vi "Get Library Icon.vi"(8 "error in (no error)":errorcluster, 11 "Library Refnum in":refnum<vi>) -> (0 "error out":errorcluster, 2 "Icon":refnum<class "Icon.lvclass">, 3 "Library Refnum out":refnum<vi>)   [LabVIEW 2017, in "LabVIEW Icon API.lvlib"]
doc: "Returns the LabVIEW Icon class of the Library.\nIf the Library doesn't have any stored data, the default LabVIEW Icon class is returned instead."
uses:
  <vilib>/LabVIEW Icon API/LabVIEW Icon API.lvlib
  <vilib>/LabVIEW Icon API/lv_icon/Classes/Icon/Icon.lvclass
  <vilib>/LabVIEW Icon API/lv_icon/Controls/BodyText.ctl
  <vilib>/LabVIEW Icon API/lv_icon/Controls/Font.ctl
  <vilib>/LabVIEW Icon API/lv_icon/Controls/Alignment.ctl
  <vilib>/LabVIEW Icon API/lv_icon/lv_icon.lvlib
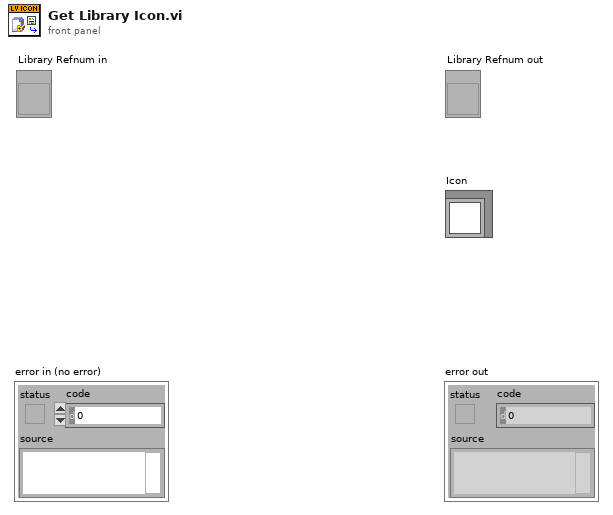
[diagram p1: front panel]
types:
  T1 = typedef "BodyText.ctl" = cluster{"Line 1 text":string, "Line 2 text":string, "Line 3 text":string, "Line 4 text":string, "Line 1 color":u32, "Line 2 color":u32, "Line 3 color":u32, "Line 4 color":u32, "Body Text Spec":cluster{"Font":T2, "Alignment":T3, "Size":u8}, "Center text vertically":bool, "Capitalize Text":bool}
  T2 = typedef "Font.ctl" = string
  T3 = typedef "Alignment.ctl" = u16
  T4 = typedef "LabVIEW Icon Stored Information.ctl" = cluster{"Text Visible?":bool, "Text Opacity":u8, "Templ Visible?":bool, "Templ Opacity":u8, "Relative Path from 1 to 2":path, "Image":picture, "All User Layers":refnum<class "Layer.lvclass">[], "Body Text":T1}
  T5 = typedef "imagedata.ctl" = cluster{"image type":i32, "image depth":i32, "image":u8[], "mask":u8[], "colors":u32[], "Rectangle":cluster{"left":i16, "top":i16, "right":i16, "bottom":i16}}
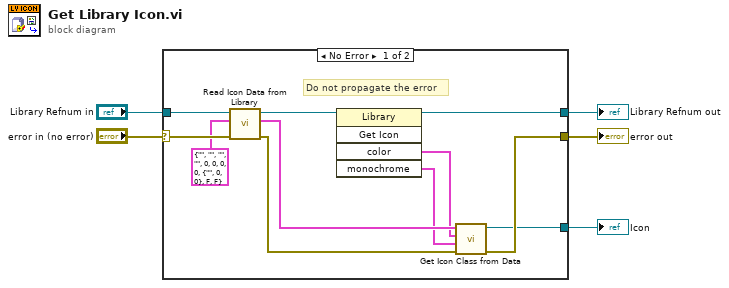
[diagram p0: block diagram]
diagram:
  n1 = case shown="No Error" "error in (no error)" {
    selector: "error in (no error)" -> [w16 w17]
    tunnel: [w12 w17] -> w4
    tunnel: "Library Refnum in" -> [w15 w18]
    tunnel: [w8 w18] -> w2
    tunnel: [w11 _] -> w1
    frame No Error {
      # "Do not propagate the error"
      n2 = call <vilib>:"Read Icon Data from Library.vi"("error in (no error)"=w16, "Default body text"=T1 {"Line 1 text"="", "Line 2 text"="", "Line 3 text"="", "Line 4 text"="", "Line 1 color"=0, "Line 2 color"=0, "Line 3 color"=0, "Line 4 color"=0, "Body Text Spec"={"Font"="", "Alignment"=0, "Size"=0}, "Center text vertically"=FALSE, "Capitalize Text"=FALSE}, "Library in"=w15) -> ("error out"=w13:errorcluster, "Data"=w9:T4, "Library out"=w10:refnum<vi>)  [unwired: 6 in]
      n3 = invoke class="Library" method="Get Icon"(reference=w10) -> (reference out=w8:refnum<vi>, "color"=w7:T5, "monochrome"=w6:T5)  [unwired: 4 in, 2 out]
      n4 = call <vilib>:"Get Icon Class from Data.vi"("error in (no error)"=w13, "BW Icon"=w6, "Color Icon"=w7, "Icon Data"=w9) -> ("error out"=w12:errorcluster, "Icon out"=w11:refnum<class "Icon.lvclass">)  [unwired: 6 in]
    }
    frame Error {
    }
  }
  "error out" <- w4
  "Icon" <- w1
  "Library Refnum out" <- w2
